vi "MeasuringDevice.Measure.vi"(8 "error in (no error)":errorcluster, 11 "LIA":refnum<class "LIA.lvclass">) -> (0 "error out":errorcluster, 2 "Result":variant, 3 "LIA out":refnum<class "LIA.lvclass">)   [LabVIEW 2017, in "LIA.lvclass"]
doc: "---------------------------------------------------------------\nJKI State Machine Objects™\nhttp://jki.net/state-machine-objects/\nCopyright (C) 2005-2015, JKI <info@jki.net>\nALL RIGHTS RESERVEDJKI State Machine Objects (SMO) 1.0.0.5\nJKI - JKI\nCopyright (c) 2016, JKI"
uses:
  LIA.lvclass
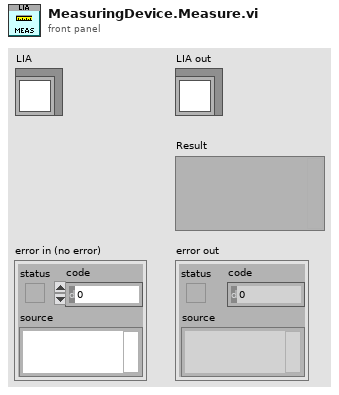
[diagram p1: front panel]
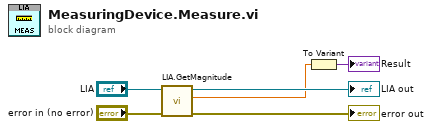
[diagram p0: block diagram]
diagram:
  n1 = call-dynamic "LIA.GetMagnitude.vi"("error in (no error)"="error in (no error)", "LIA in"="LIA") -> ("error out"=→"error out":errorcluster, "Magnitude"=w1:dbl, "LIA out"=→"LIA out":refnum<class "LIA.lvclass">)  [unwired: 7 in]
  n2 = To Variant(anything=w1) -> (Variant=→"Result":variant)
